vi "CIPC DAQ FIFO.vi"() -> (3 "CIF_CIPC_Fifo_DAQ.lvclass":refnum<class "CIF_CIPC_Fifo_DAQ.lvclass">)   [LabVIEW 2021, in "CIF_CIPC_Fifo_DAQ.lvclass"]
uses:
  CIF_CIPC_Fifo_DAQ.lvclass
  CIF_CIPC_Fifo_DAQ.lvclass/CIF_CIPC_Fifo_DAQ.ctl
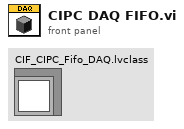
[diagram p1: front panel]
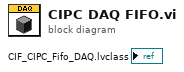
[diagram p0: block diagram]
diagram:
